vi "LV SCISDK Read Oscilloscope Dual Data.vi"(0 "Path":string, 2 "handle":u64, 3 "error in (no error)":errorcluster) -> (7 "function return":i32, 8 "buffer out":T1, 9 "handle out":u64, 10 "error out":errorcluster)   [LabVIEW 2021, in "SciSDK_Labview.lvlib"]
doc: "You need this VI to call native dll method to read data from an oscilloscope dual component"
uses:
  SciSDK_Labview.lvlib
panel:
  in  "buffer":T1
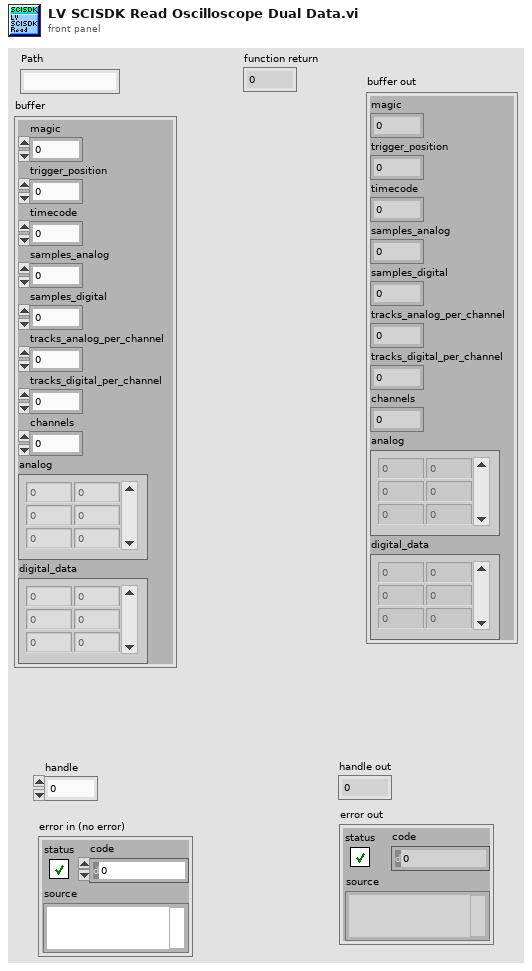
[diagram p1: front panel]
types:
  T1 = cluster{"magic":u32, "trigger_position":u32, "timecode":u32, "samples_analog":u32, "samples_digital":u32, "tracks_analog_per_channel":u32, "tracks_digital_per_channel":u32, "channels":u32, "analog":i32[][], "digital_data":i32[][]}
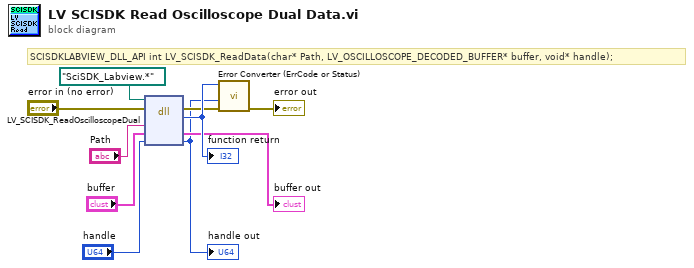
[diagram p0: block diagram]
diagram:
  # "SCISDKLABVIEW_DLL_API int LV_SCISDK_ReadData(char* Path, LV_OSCILLOSCOPE_DECODED_BUFFER* buffer, void* handle);"
  n1 = dll-call lib="C:/git/scisdk/SciSDK_VC++/x64/Debug/SciSDK_Labview.dll" fn="LV_SCISDK_ReadOscilloscopeDual"(path in=path "SciSDK_Labview.*", error in="error in (no error)", "Path"="Path", "buffer"="buffer", "handle"="handle") -> (error out=w6:errorcluster, "return type"=w10:i32, "buffer"=→"buffer out":T1, "handle"=w1:u64)  [unwired: 2 in, 1 out]
  "function return" <- w10
  "handle out" <- w1
  n2 = call "Error Converter (ErrCode or Status).vi"("error in (no error)"=w6, "handle"=w1, "error code"=w10) -> ("error out"=→"error out":errorcluster)  [unwired: 8 in]
